vi "Write Level.vi"(8 "error in (no error)":errorcluster, 10 "Level":T1={"InputImpedance"=0.0, "AttenuationAuto"=FALSE, "ReferenceLevel"=0.0, "Attenuation"=0.0, "ReferenceLevelOffset"=0.0, "amplitude units (dBm)"=1} {"amplitude units (dBm)" items=["dBm"=1, "dBmV"=2, "dBuV"=3, "dBuA"=1001, "Volt"=4, "Watt"=5, "Amper"=1002]}, 11 "SpecAnBase in":refnum<class "SpecAnBase.lvclass">) -> (0 "error out":errorcluster, 3 "SpecAnBase out":refnum<class "SpecAnBase.lvclass">)   [LabVIEW 2018, in "SpecAnPlugins.lvlib" / "SpecAnBase.lvclass"]
uses:
  SpecAnBase.lvclass
  Typedefs/Level.ctl
  SpecAnBase.lvclass/SpecAnBase.ctl
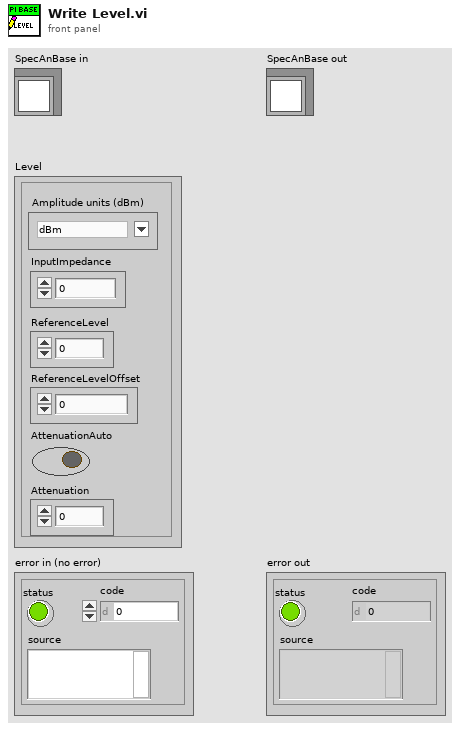
[diagram p1: front panel]
types:
  T1 = typedef "SpecAnPlugins.lvlib/SpecAnBase.lvclass/Level.ctl" = cluster{"InputImpedance":dbl, "AttenuationAuto":bool, "ReferenceLevel":dbl, "Attenuation":dbl, "ReferenceLevelOffset":dbl, "amplitude units (dBm)":i32}
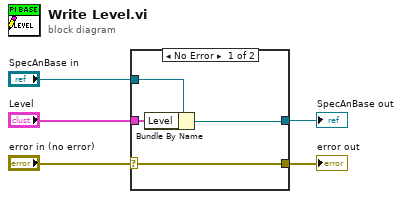
[diagram p0: block diagram]
diagram:
  n1 = case shown="No Error" "error in (no error)" {
    selector: "error in (no error)" -> [w9 w10]
    tunnel: [w9 w10] -> w4
    tunnel: [w7 w11] -> w2
    tunnel: "SpecAnBase in" -> [w8 w11]
    tunnel: "Level" -> [w6 _]
    frame No Error {
      n2 = Bundle By Name(cluster=w8, "Level"=w6) -> (w7:refnum<class "SpecAnBase.lvclass">)
    }
    frame Error {
    }
  }
  "error out" <- w4
  "SpecAnBase out" <- w2
